vi "test1.vi"() -> ()   [LabVIEW 2020]
panel:
  in  "布尔 4":bool
  out "布尔 3":bool=TRUE
  out "Class Hierarchy":string[](array[string]) caption="类层次结构"
  out "布尔":bool
  in  "小尾寒羊t":bool
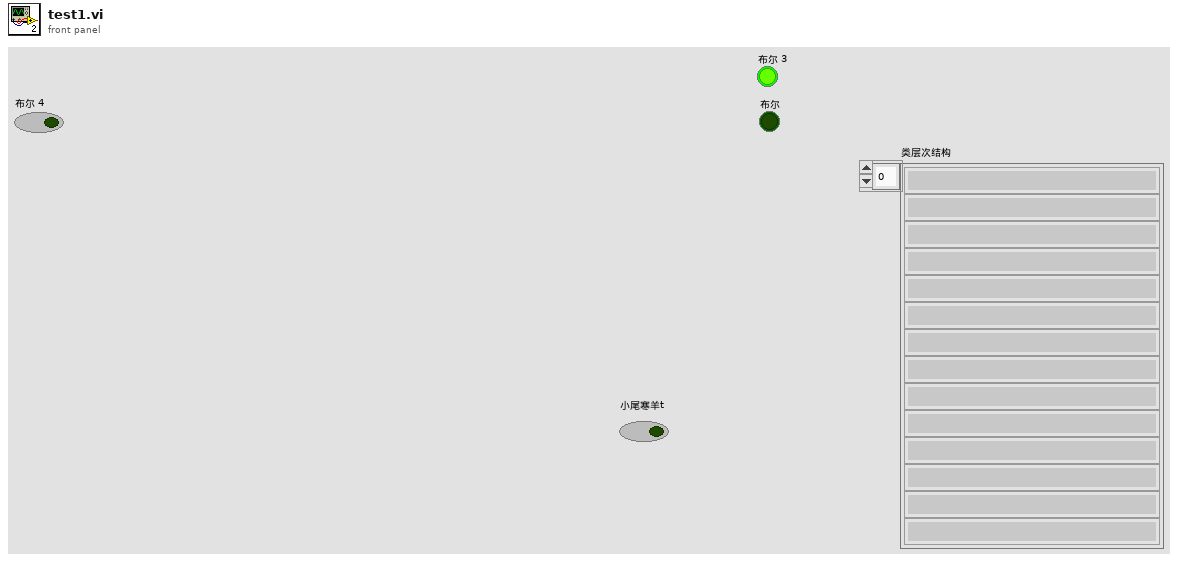
[diagram p1: front panel]
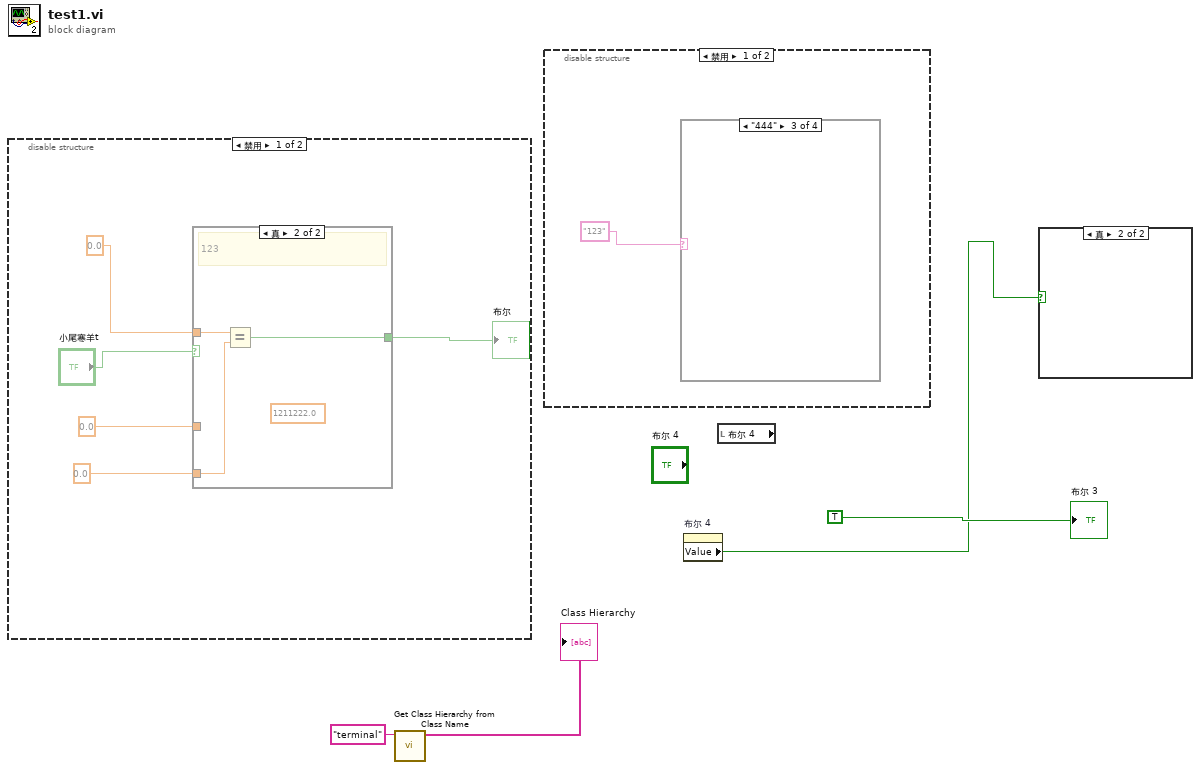
[diagram p0: block diagram]
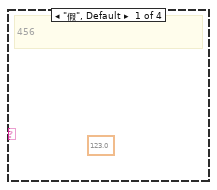
[diagram p3: hidden frame]
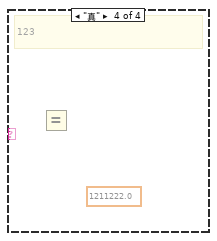
[diagram p5: hidden frame]
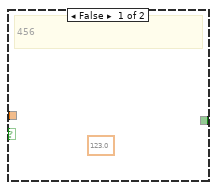
[diagram p7: hidden frame]
diagram:
  n1 = disable-structure shown="禁用" {
    frame Disabled {
      n2 = case shown="真" "小尾寒羊t" {
        tunnel: 0.0 -> [_ w12]
        tunnel: 0.0 -> [_ w11]
        tunnel: [_ w10] -> w6
        tunnel: 0.0 -> [_ _]
        frame False {
          (unwired) 123.0
          # "456"
        }
        frame True {
          (unwired) 1211222.0
          # "123"
          n3 = Equal?(x=w12, y=w11) -> (x = y?=w10:bool)
        }
      }
      "布尔" <- w6
    }
    frame Enabled {
    }
  }
  n4 = call <vilib>:"Get Class Hierarchy from Class Name.vi"("Class Name"="terminal") -> ("Class Hierarchy"=→"Class Hierarchy":string[])  [unwired: 9 in, 1 out]
  n5 = disable-structure shown="禁用" {
    frame Disabled {
      n6 = case shown="\"444\"" "123" {
        frame "假", Default {
          (unwired) 123.0
          # "456"
        }
        frame "123" {
        }
        frame "444" {
        }
        frame "真" {
          (unwired) 1211222.0
          # "123"
          n7 = Equal?() -> ()  [unwired: 2 in, 1 out]
        }
      }
    }
    frame Enabled {
    }
  }
  n8 = property on="布尔 4" class="Bool (严格)"() -> ("Value"=w1:bool)  [unwired: 2 in, 2 out]
  n9 = local read "布尔 4"() -> ()  [unwired: 1 out]
  n10 = case shown="真" w1 {
    frame False {
    }
    frame True {
    }
  }
  "布尔 3" <- TRUE
